vi "Scope_V1.vi"(9 "ObjectChoice":i32[](listbox), 11 "btnSelectObject":bool) -> (0 "strObjectDispArray":string[](array[string]), 1 "mu08ArrayIndexFinalOut":u8[](array[numeric]), 2 "NamePic":picture, 3 "mbfObjectChoiceArray":bool[](array[boolean]))   [LabVIEW 2011]
uses:
  <vilib>/Utility/miscctls.llb/LVPoint32TypeDef.ctl
  GlobalVariable/strGlobalVariable.vi
panel:
  out "Chart":T1(graph) caption="带状图表（2条曲线，每次更新1个点）"
  out "strArrayOut":string[](array[string])
  out "mu32ArrayOut":u32[](array[numeric])
  out "mbfStartDraw":bool
  out "btnSelectObject.Txt":string
  out "坐标":T2
  out "mu08ObjectArraySize":u8
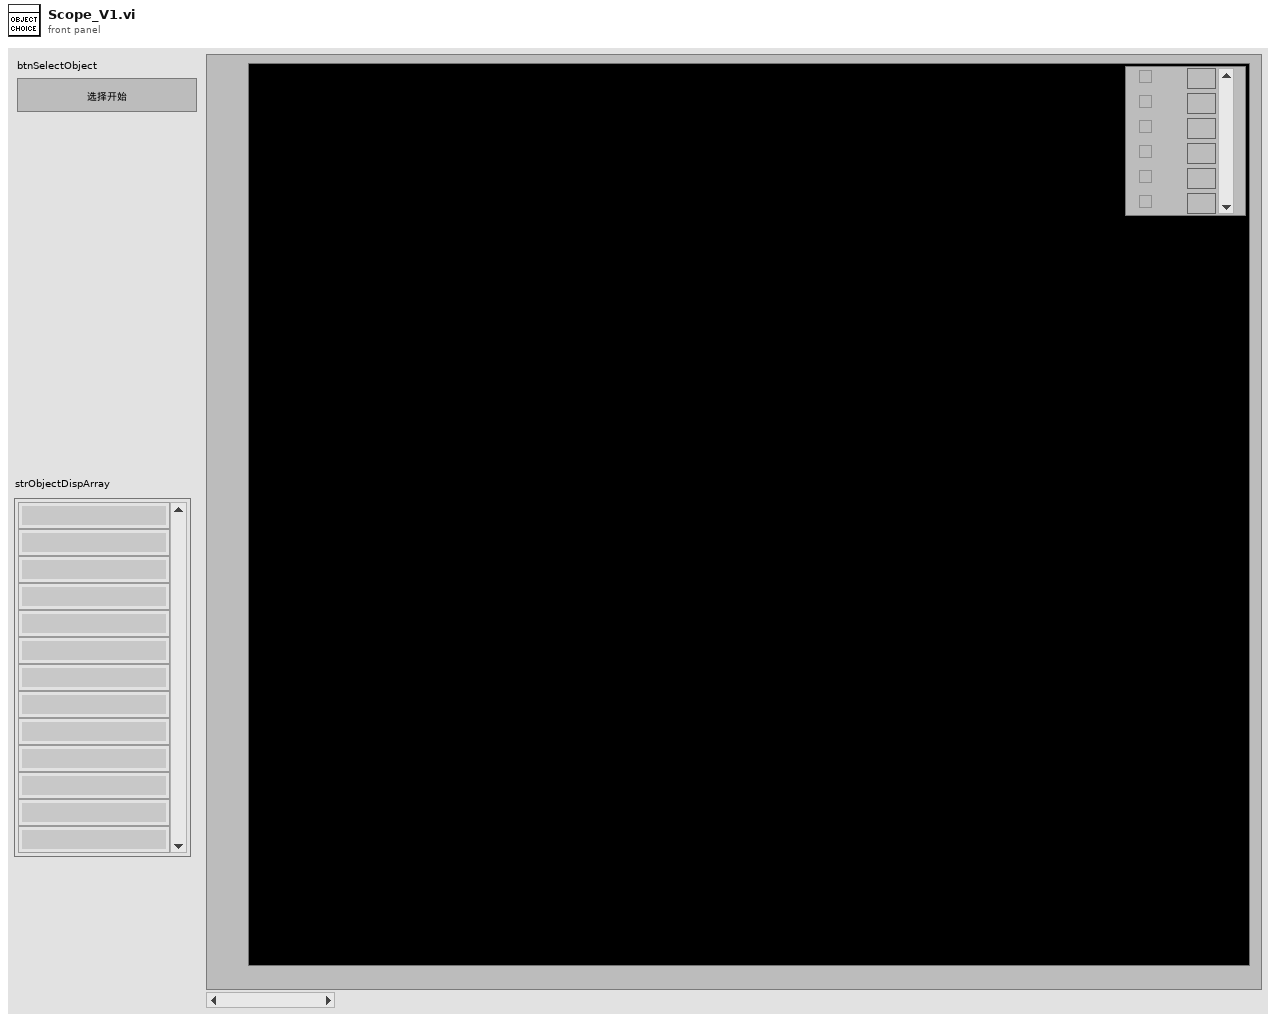
[diagram p1: front panel]
types:
  T1 = cluster{"Value[0]":u32, "Value[1]":u32, "Value[2]":u32, "Value[3]":u32, "Value[4]":u32, "Value[5]":u32, "Value[6]":u32, "Value[7]":u32, "Value[8]":u32}
  T2 = typedef "LVPoint32TypeDef.ctl" = cluster{"Horizontal":i32, "Vertical":i32}
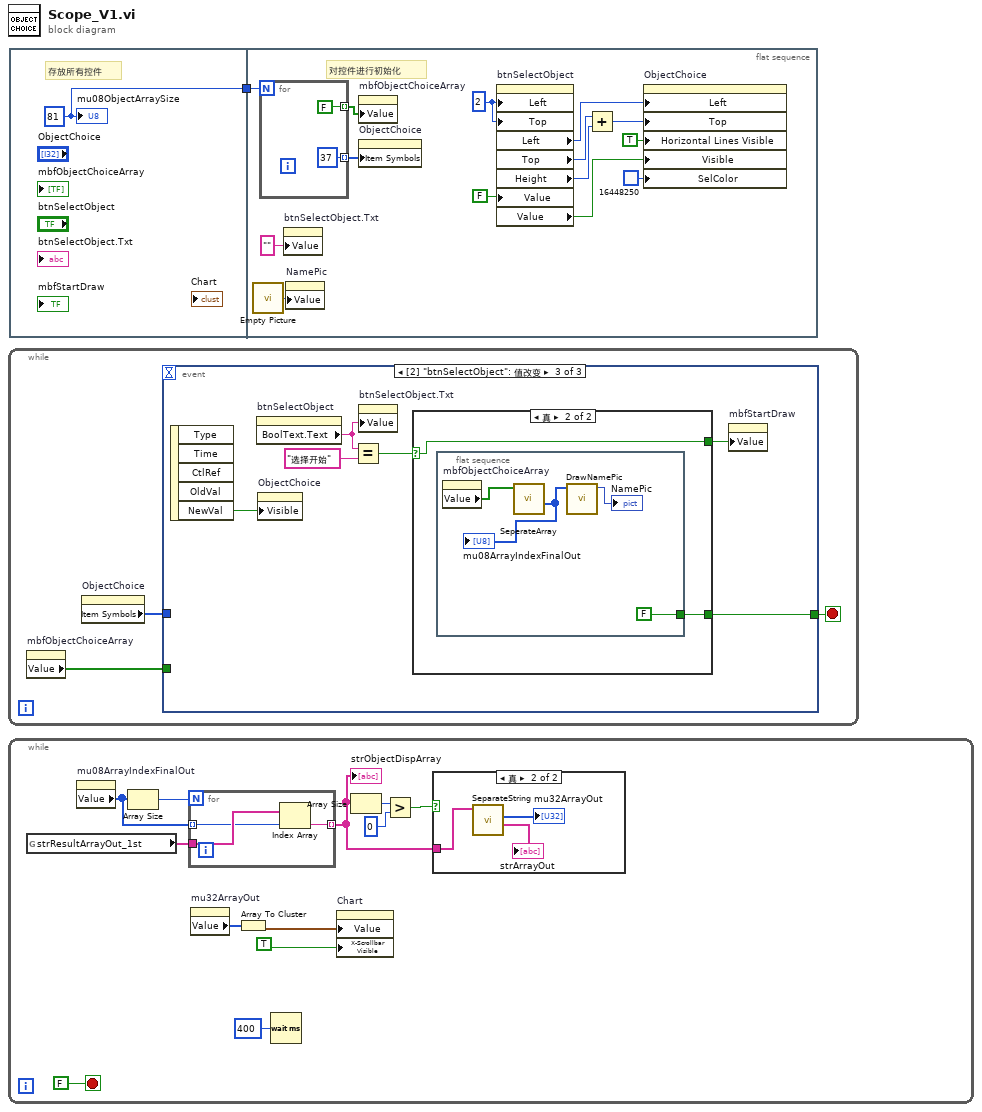
[diagram p0: block diagram]
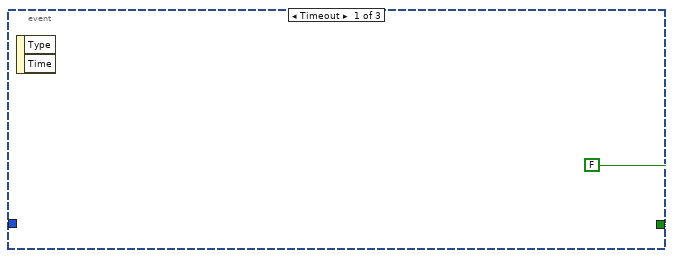
[diagram p3: hidden frame]
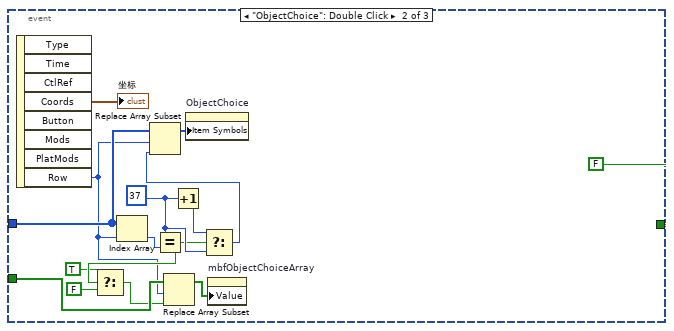
[diagram p4: hidden frame]
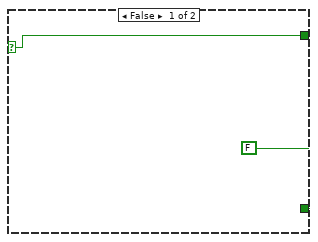
[diagram p5: hidden frame]
diagram:
  n1 = while {
    stop <- w2 stop-if-true
    n2 = property on="mbfObjectChoiceArray" class="Arr (严格)"() -> ("Value"=w3:bool[])  [unwired: 2 in, 2 out]
    n3 = property on="ObjectChoice" class="LstBox (严格)"() -> ("Item Symbols"=w4:i32[])  [unwired: 2 in, 2 out]
    n4 = event shown="[2] \"btnSelectObject\": 值改变" {
      selector: _ -> [_ _ _]
      dyn-events: _ -> [_ _ _]
      timeout: _ -> [_ _ _]
      tunnel: w4 -> [_ w19 _]
      tunnel: w3 -> [_ w10 _]
      tunnel: [FALSE FALSE w21] -> w2
      event Timeout {
        n5 = event-data() -> ()  [unwired: 1 in, 2 out]
      }
      event "ObjectChoice": Double Click {
        w15 = 37 ("y")
        n6 = event-data() -> ("Coords"=→"坐标":T2, "Row"=w7:i32)  [unwired: 1 in, 6 out]
        n7 = Index Array(array=w19, index=w7) -> (element=w17:i32)
        n8 = Equal?(x=w15, y=w17) -> (x = y?=w13:bool)
        n9 = Select(t=TRUE, s=w13, f=FALSE) -> (s? t:f=w9:bool)
        n10 = Replace Array Subset(array=w10, new element=w9, index=w7) -> (w8:bool[])
        n11 = Increment(x=w15) -> (x+1=w16:i32)
        n12 = Select(t=w16, s=w13, f=w15) -> (s? t:f=w14:i32)
        n13 = Replace Array Subset(array=w19, new element=w14, index=w7) -> (w18:i32[])
        n14 = property on="ObjectChoice" class="LstBox (严格)"("Item Symbols"=w18) -> ()  [unwired: 2 in, 2 out]
        n15 = property on="mbfObjectChoiceArray" class="Arr (严格)"("Value"=w8) -> ()  [unwired: 2 in, 2 out]
      }
      event "btnSelectObject": Value Change {
        n16 = event-data() -> ("NewVal"=w26:bool)  [unwired: 1 in, 4 out]
        n17 = property on="btnSelectObject" class="Bool (严格)"() -> ("BoolText.Text"=w25:string)  [unwired: 2 in, 2 out]
        n18 = property on="ObjectChoice" class="LstBox (严格)"("Visible"=w26) -> ()  [unwired: 2 in, 2 out]
        n19 = Equal?(x=w25, y="选择开始") -> (x = y?=w23:bool)
        n20 = property on="btnSelectObject.Txt" class="Str"("Value"=w25) -> ()  [unwired: 2 in, 2 out]
        n21 = case shown="真" w23 {
          selector: w23 -> [w28 w30]
          tunnel: [w28 w30] -> w22
          tunnel: [FALSE w29] -> w21
          frame False {
          }
          frame True {
            n22 = flat-sequence {
              tunnel: [FALSE] -> w29
              frame #0 {
                n23 = property on="mbfObjectChoiceArray" class="Arr (严格)"() -> ("Value"=w34:bool[])  [unwired: 2 in, 2 out]
                n24 = call "SeperateArray.vi"("mbfArrayIn"=w34) -> ("mu08ArrayIndexFinalOut"=w31:u8[])  [unwired: 9 in, 1 out]
                "mu08ArrayIndexFinalOut" <- w31
                n25 = call "DrawNamePic.vi"("mu08ArrayIn"=w31) -> ("NamePic"=→"NamePic":picture)  [unwired: 10 in]
              }
            }
          }
        }
        n26 = property on="mbfStartDraw" class="Bool (严格)"("Value"=w22) -> ()  [unwired: 2 in, 2 out]
      }
    }
  }
  n27 = while {
    stop <- FALSE stop-if-true
    n28 = global read "strGlobalVariable.vi" "strResultArrayOut_1st"() -> (w45:string[])
    n29 = property on="mu08ArrayIndexFinalOut" class="Arr (严格)"() -> ("Value"=w44:u8[])  [unwired: 2 in, 2 out]
    n30 = Array Size(array=w44) -> (size(s)=w39:i32)
    n31 = for {
      N: w39 -> [_]
      tunnel: w45 -> [w52]
      tunnel: w44 -> [w51] mode=indexing
      tunnel: [w50] -> w40 mode=indexing
      n32 = Index Array(array=w52, index=w51) -> (element=w50:string)
    }
    "strObjectDispArray" <- w40
    n33 = property on="mu32ArrayOut" class="Arr (严格)"() -> ("Value"=w38:u32[])  [unwired: 2 in, 2 out]
    n34 = Array To Cluster(array=w38) -> (cluster=w37:T1)
    n35 = Wait (ms)(milliseconds to wait=u32 400 ("等待时间（毫秒）")) -> ()  [unwired: 1 out]
    n36 = property on="Chart" class="WFChart (严格)"("Value"=w37, "X-Scrollbar Visible"=TRUE ("X滚动条可见")) -> ()  [unwired: 2 in, 2 out]
    n37 = Array Size(array=w40) -> (size(s)=w43:i32)
    n38 = Greater?(x=w43, y=0) -> (0:w41:bool)
    n39 = case shown="真" w41 {
      tunnel: w40 -> [_ w49]
      frame False {
      }
      frame True {
        n40 = call "SeparateString.vi"("strArrayIn"=w49) -> ("strArrayOut"=→"strArrayOut":string[], "mu32ArrayOut"=→"mu32ArrayOut":u32[])  [unwired: 8 in, 1 out]
      }
    }
  }
  n41 = flat-sequence {
    tunnel: [w53] -> w1
    tunnel: w1 -> [w67]
    frame #0 {
      w53 = u8 81 ("mu08ObjectArraySize")
      # "存放所有控件"
      "mu08ObjectArraySize" <- w53
    }
    frame #1 {
      w59 = 2 ("位置:居左")
      # "对控件进行初始化"
      n42 = call "Empty Picture"() -> ("empty picture"=w54:picture)
      n43 = for {
        N: w67 -> [_]
        tunnel: [FALSE] -> w65 mode=indexing
        tunnel: [37] -> w66 mode=indexing
      }
      n44 = property on="btnSelectObject.Txt" class="Str"("Value"="" ("btnSelectObject.Txt")) -> ()  [unwired: 2 in, 2 out]
      n45 = property on="NamePic" class="Pict"("Value"=w54) -> ()  [unwired: 2 in, 2 out]
      n46 = property on="mbfObjectChoiceArray" class="Arr (严格)"("Value"=w65) -> ()  [unwired: 2 in, 2 out]
      n47 = property on="ObjectChoice" class="LstBox (严格)"("Item Symbols"=w66) -> ()  [unwired: 2 in, 2 out]
      n48 = property on="btnSelectObject" class="Bool (严格)"("Left"=w59, "Top"=w59, "Value"=FALSE ("btnSelectObject")) -> ("Left"=w64:i32, "Top"=w57:i32, "Height"=w63:u32, "Value"=w58:bool)  [unwired: 2 in, 2 out]
      n49 = Add(x=w57, y=w63) -> (x+y=w62:u32)
      n50 = property on="ObjectChoice" class="LstBox (严格)"("Left"=w64, "Top"=w62, "Horizontal Lines Visible"=TRUE, "Visible"=w58, "SelColor"=u32 16448250) -> ()  [unwired: 2 in, 2 out]
    }
  }
